vi "_CreacionArchivos.vi"(9 "Tipo_Data":string, 10 "Nombre_mision":string, 11 "Carpeta":string) -> (3 "appended path":path)   [LabVIEW 2018]
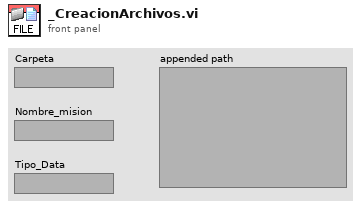
[diagram p1: front panel]
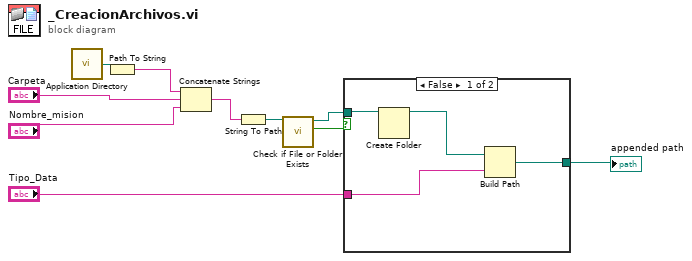
[diagram p0: block diagram]
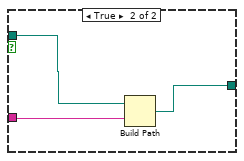
[diagram p2: hidden frame]
diagram:
  n1 = call <vilib>:"Application Directory.vi"() -> ("Application Directory"=w1:path)
  n2 = Path To String(path=w1) -> (string=w3:string)
  n3 = Concatenate Strings(w3, "Carpeta", "Nombre_mision") -> (w4:string)
  n4 = String To Path(string=w4) -> (path=w5:path)
  n5 = call <vilib>:"Check if File or Folder Exists.vi"("path"=w5) -> ("file or folder exists?"=w6:bool, "dup path"=w7:path)  [unwired: 8 in, 1 out]
  n6 = case shown="False" w6 {
    tunnel: w7 -> [w13 w17]
    tunnel: [w12 w16] -> w9
    tunnel: "Tipo_Data" -> [w11 w15]
    frame False {
      n7 = Create Folder(path (use dialog)=w13) -> (created path=w14:path)  [unwired: 2 in, 2 out]
      n8 = Build Path(base path=w14, name or relative path=w11) -> (appended path=w12:path)
    }
    frame True {
      n9 = Build Path(base path=w17, name or relative path=w15) -> (appended path=w16:path)
    }
  }
  "appended path" <- w9
